vi "chart series set points.vi"(8 "error in (no error)":errorcluster, 10 "points":u32, 11 "series":u32) -> (0 "error out":errorcluster, 3 "function return":u32(ring))   [LabVIEW 8.6]
doc: "lxw_error chart_series_set_points(lxw_chart_series series, unsigned long points);"
uses:
  pending_lvxlsxwriter/xlsxwriter.dll
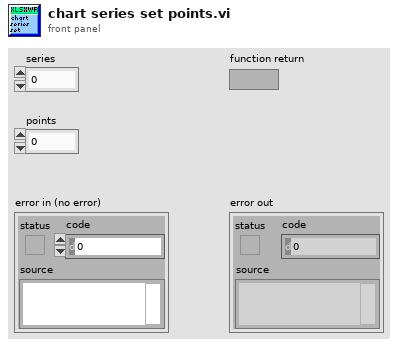
[diagram p1: front panel]
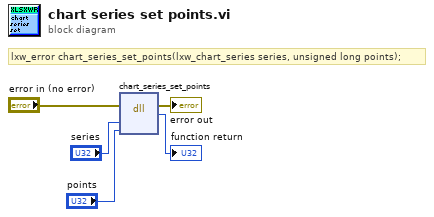
[diagram p0: block diagram]
diagram:
  # "lxw_error chart_series_set_points(lxw_chart_series series, unsigned long points);"
  n1 = dll-call lib="C:/Users/WDAGUtilityAccount/Desktop/pending_lvxlsxwriter/xlsxwriter.*" fn="chart_series_set_points"(error in="error in (no error)", "series"="series", "points"="points") -> (error out=→"error out":errorcluster, →"function return":u32)  [unwired: 4 in, 1 out]
